vi "TechnicalTest.vi"() -> ()   [LabVIEW 2020]
panel:
  in  "Input Sensor Value":dbl
  out "Last 5 Average":dbl
  out "Action":string
  out "Values":dbl[](array[numeric])
  in  "stop":bool
  in  "Read Sensor":bool
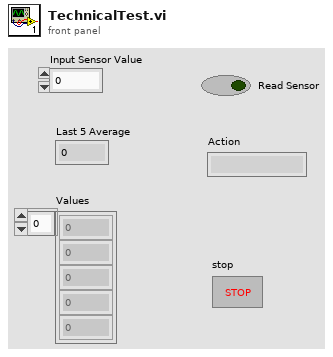
[diagram p1: front panel]
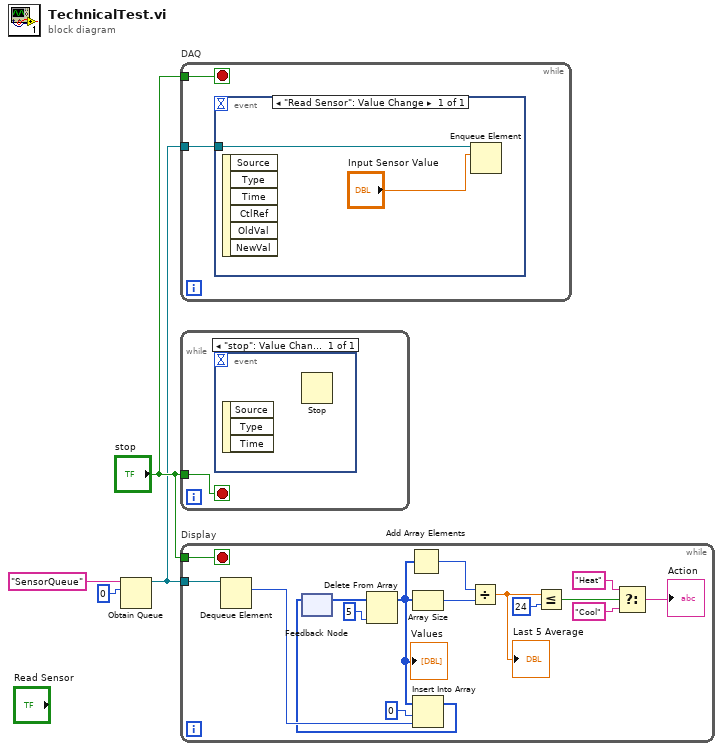
[diagram p0: block diagram]
diagram:
  n1 = Obtain Queue(name (unnamed)="SensorQueue", element data type=0) -> (queue out=w2:refnum<queue>)  [unwired: 3 in, 2 out]
  n2 = while "DAQ" {
    tunnel: w2 -> [w6]
    tunnel: "stop" -> [w5]
    stop <- w5 stop-if-true
    n3 = event shown="[0] \"Read Sensor\": Value Change" {
      selector: _ -> [_]
      dyn-events: _ -> [_]
      timeout: _ -> [_]
      tunnel: w6 -> [w8]
      event "Read Sensor": Value Change {
        n4 = event-data() -> ()  [unwired: 1 in, 6 out]
        n5 = Enqueue Element(queue=w8, element="Input Sensor Value") -> ()  [unwired: 2 in, 3 out]
      }
    }
  }
  n6 = while {
    tunnel: "stop" -> [w9]
    stop <- w9 stop-if-true
    n7 = event shown="[0] \"stop\": Value Change" {
      selector: _ -> [_]
      dyn-events: _ -> [_]
      timeout: _ -> [_]
      event "stop": Value Change {
        n8 = event-data() -> ()  [unwired: 1 in, 3 out]
        n9 = Stop() -> ()  [unwired: 1 in]
      }
    }
  }
  n10 = while "Display" {
    tunnel: w2 -> [w23]
    tunnel: "stop" -> [w10]
    stop <- w10 stop-if-true
    n11 = Dequeue Element(queue=w23) -> (element=w17:i32)  [unwired: 2 in, 3 out]
    n12 = feedback #1() -> (w14:i32[])  [unwired: 1 in]
    n13 = Delete From Array(array=w14, index=5) -> (array with subset deleted=w12:i32[])  [unwired: 1 in, 1 out]
    "Values" <- w12
    n14 = Add Array Elements(numeric array=w12) -> (sum=w24:i32)
    n15 = Array Size(array=w12) -> (size(s)=w11:i32)
    n16 = Insert Into Array(array=w12, index=0, new element=w17) -> (w15:i32[])
    n17 = feedback-in #1(w15) -> ()
    n18 = Divide(x=w24, y=w11) -> (x/y=w16:dbl)
    "Last 5 Average" <- w16
    n19 = Less Or Equal?(x=w16, y=24) -> (x <= y?=w19:bool)
    n20 = Select(t="Heat", s=w19, f="Cool") -> (s? t:f=→"Action":string)
  }
